vi "InsertValuesIntoSp.vi"() -> ()   [LabVIEW 2019]
uses:
  <vilib>/addons/database/NI_Database_API.lvlib
  <vilib>/addons/database/Connection.llb/DB Tools Open Connec (String).vi
  <vilib>/addons/database/Connection.llb/Conn Execute.vi
panel:
  out "PassFail":bool
  in  "Subject  Name":string
  in  "?":dbl
  # "Marks"
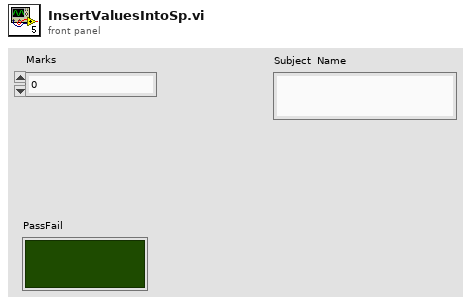
[diagram p1: front panel]
types:
  T1 = typedef "NI_Database_API.lvlib/Conn ObjectReference.ctl" = refnum<k1>
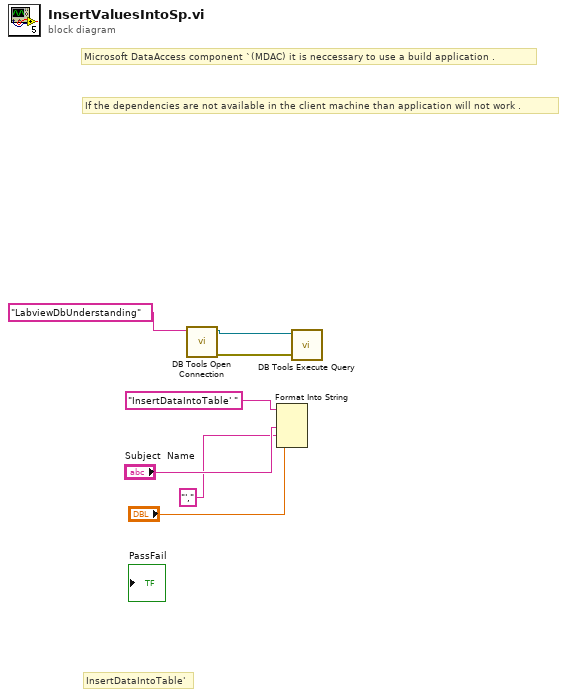
[diagram p0: block diagram]
diagram:
  # "InsertDataIntoTable'"
  # "If the dependencies are not available in the client machine than application will not work ."
  # "Microsoft DataAccess component `(MDAC) it is neccessary to use a build application ."
  n1 = call-poly <vilib>:"DB Tools Open Connection.vi"("connection information"="LabviewDbUnderstanding") -> ("error out"=w5:errorcluster, "connection reference"=w6:T1)  [unwired: 7 in]
  n2 = Format Into String(initial string="InsertDataIntoTable' ", "Subject  Name", "',", "?") -> ()  [unwired: 2 in, 2 out]
  n3 = call-poly <vilib>:"DB Tools Execute Query.vi"("error in (no error)"=w5, "connection reference"=w6) -> ()  [unwired: 6 in, 2 out]
